vi "OscopeSession.vi"(8 "Session In":refnum<class "Device Session.lvclass">, 9 "Bitfile Path In":string, 10 "Device Address In":string, 11 "Write":bool) -> (0 "Session Out":refnum<class "Device Session.lvclass">, 1 "Bitfile Path Out":string, 2 "Device Address Out":string)   [LabVIEW 2015]
uses:
  OscopeAPI/Device Session.lvclass
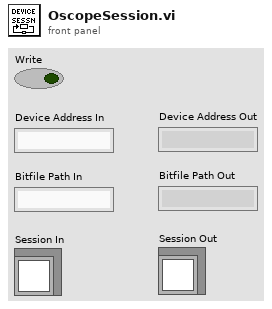
[diagram p1: front panel]
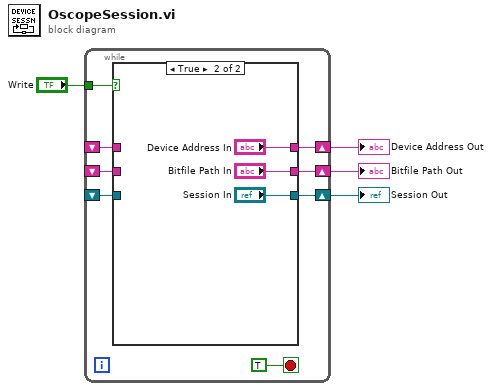
[diagram p0: block diagram]
diagram:
  n1 = while {
    tunnel: "Write" -> [w11]
    shift-right: [w10] -> w3
    shift-left: _ -> [w9]
    shift-right: [w8] -> w2
    shift-left: _ -> [w7]
    shift-right: [w6] -> w1
    shift-left: _ -> [w5]
    stop <- TRUE stop-if-true
    n2 = case shown="True" w11 {
      tunnel: [w15 "Device Address In"] -> w10
      tunnel: w9 -> [w15 _]
      tunnel: [w14 "Bitfile Path In"] -> w8
      tunnel: w7 -> [w14 _]
      tunnel: [w13 "Session In"] -> w6
      tunnel: w5 -> [w13 _]
      frame False {
      }
      frame True {
      }
    }
  }
  "Device Address Out" <- w3
  "Bitfile Path Out" <- w2
  "Session Out" <- w1
